vi "VCS Digital Output Configuration.vi"(8 "error in (no error)":errorcluster, 10 "output configuration":T1={"digitalOutputNumber"=1, "configuration"=0, "state"=0, "mask"=0, "polarity"=0} {"polarity" items=["high active", "low active"]; "mask" items=["disabled", "enabled"]; "state" items=["inactive", "active"]; "configuration" items=["ready"=0, "position compare"=1, "general purpose A"=15, "general purpose B"=14, "general purpose C"=13, "general purpose D"=12, "general purpose E"=11, "general purpose F"=10, "general purpose G"=9, "general purpose H"=8]}, 11 "axis in":cluster{"keyHandle":u32, "nodeId":u16}={"keyHandle"=0, "nodeId"=1}) -> (0 "error out":errorcluster, 3 "axis out":cluster{"keyHandle":u32, "nodeId":u16}={"keyHandle"=0, "nodeId"=1})   [LabVIEW 2018]
doc: "<B>VCS Digital Output Configuration</B> sets parameter for one digital output."
uses:
  Resources/EposCmd.dll
  Resources/EposCmd64.dll
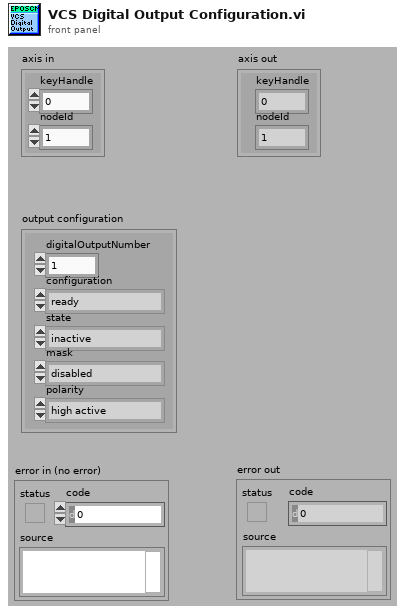
[diagram p1: front panel]
types:
  T1 = cluster{"digitalOutputNumber":u16, "configuration":u16, "state":i32, "mask":i32, "polarity":i32}
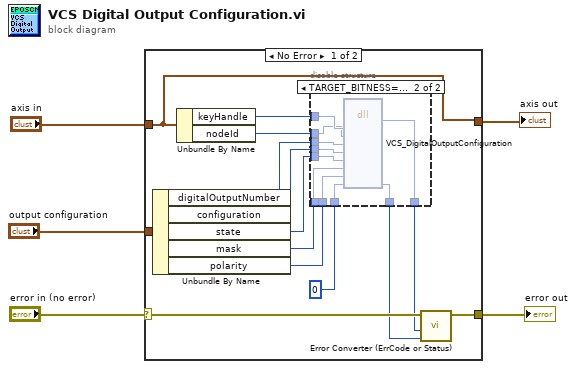
[diagram p0: block diagram]
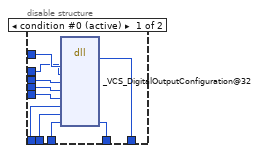
[diagram p2: hidden frame]
diagram:
  n1 = case shown="No Error" "error in (no error)" {
    selector: "error in (no error)" -> [w19 w41]
    tunnel: [w18 w41] -> w4
    tunnel: "axis in" -> [w9 w40]
    tunnel: "output configuration" -> [w15 _]
    tunnel: [w9 w40] -> w1
    frame No Error {
      n2 = Unbundle By Name(w15) -> ("digitalOutputNumber"=w14:u16, "configuration"=w13:u16, "state"=w12:i32, "mask"=w11:i32, "polarity"=w10:i32)
      n3 = Unbundle By Name(w9) -> ("keyHandle"=w17:u32, "nodeId"=w16:u16)
      n4 = disable-structure shown="TARGET_BITNESS==64" {
        disable-tunnel: w17 -> [w29 w39]
        disable-tunnel: w16 -> [w28 w38]
        disable-tunnel: w14 -> [w27 w37]
        disable-tunnel: w13 -> [w26 w36]
        disable-tunnel: w12 -> [w25 w35]
        disable-tunnel: w11 -> [w24 w34]
        disable-tunnel: w10 -> [w23 w33]
        disable-tunnel: u32 0 ("pErrorCode") -> [w22 w32]
        disable-tunnel: [w21 w31] -> w7
        disable-tunnel: [w20 w30] -> w6
        frame condition #0 (active) {
          n5 = dll-call lib="C:/Projeto em LabVIEW/EPOS-LabVIEW-Instrument-Driver-En/LabVIEW/maxon EPOS/Resources/EposCmd.*" fn="_VCS_DigitalOutputConfiguration@32"("KeyHandle"=w29, "NodeId"=w28, "DigOutputNb"=w27, "Configuration"=w26, "State"=w25, "Mask"=w24, "Polarity"=w23, "pErrorCode"=w22) -> (w20:i32, "pErrorCode"=w21:u32)  [unwired: 10 in, 2 out]
        }
        frame condition #1 {
          n6 = dll-call lib="C:/setup/Resources/EposCmd64.*" fn="VCS_DigitalOutputConfiguration" ("EposCmd.dll:_VCS_DigitalOutputConfiguration@32")("KeyHandle"=w39, "NodeId"=w38, "DigOutputNb"=w37, "Configuration"=w36, "State"=w35, "Mask"=w34, "Polarity"=w33, "pErrorCode"=w32) -> ("Rückgabetyp"=w30:i32, "pErrorCode"=w31:u32)  [unwired: 10 in, 2 out]
        }
      }
      n7 = call "Error Converter (ErrCode or Status).vi"("error code"=w7, "return type"=w6, "error in (no error)"=w19) -> ("error out"=w18:errorcluster)  [unwired: 7 in]
    }
    frame Error {
    }
  }
  "error out" <- w4
  "axis out" <- w1
